vi "ArduinoSerialReadWrite.vi"(9 "LED":bool[](array[boolean])=[FALSE, FALSE, FALSE, FALSE, FALSE], 11 "VISA resource name":refnum<visa-resource-name>) -> (0 "error out":errorcluster, 1 "AIs":dbl[](array[numeric]), 2 "Buttons":bool[](array[boolean]), 3 "VISA resource name out":refnum<visa-resource-name>)   [LabVIEW 2014]
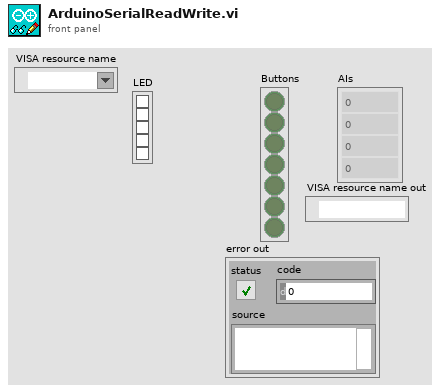
[diagram p1: front panel]
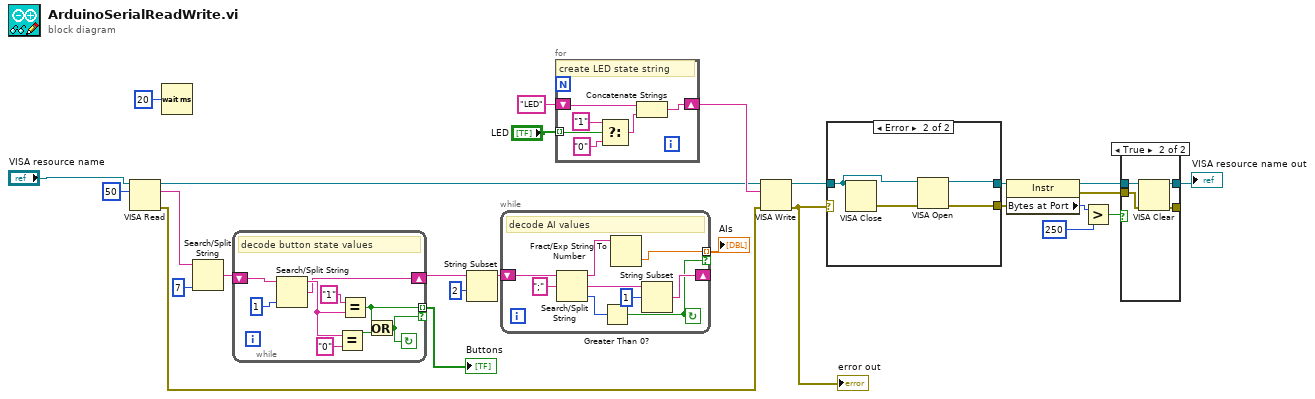
[diagram p0: block diagram]
diagram:
  n1 = VISA Read(VISA resource name="VISA resource name", byte count=u32 50) -> (VISA resource name out=w19:refnum<visa-resource-name>, read buffer=w24:string, error out=w23:errorcluster)  [unwired: 1 in, 1 out]
  n2 = Wait (ms)(milliseconds to wait=u32 20) -> ()  [unwired: 1 out]
  n3 = Search/Split String(string=w24, offset (0)=7) -> (match + rest of string=w16:string)  [unwired: 1 in, 2 out]
  n4 = while {
    tunnel: [w30] -> w15 mode=indexing if=w29
    shift-right: [w27] -> w14
    shift-left: w16 -> [w35]
    stop <- w29 continue-if-true
    # "decode button state values"
    n5 = Search/Split String(string=w35, offset (0)=1 ("length (rest)")) -> (substring before match=w28:string, match + rest of string=w27:string)  [unwired: 1 in, 1 out]
    n6 = Equal?(x=w28, y="0") -> (x = y?=w31:bool)
    n7 = Equal?(x="1" ("y"), y=w28) -> (x = y?=w30:bool)
    n8 = Or(x=w30, y=w31) -> (x .or. y?=w29:bool)
  }
  "Buttons" <- w15
  n9 = String Subset(string=w14, offset (0)=2) -> (substring=w13:string)  [unwired: 1 in]
  n10 = while {
    shift-right: [w42] -> _
    shift-left: w13 -> [w44]
    tunnel: [w38] -> w17 mode=indexing if=w37
    stop <- w37 continue-if-true
    # "decode AI values"
    n11 = Search/Split String(string=w44, search string/char (-)=";") -> (substring before match=w36:string, match + rest of string=w41:string, offset of match=w39:i32)  [unwired: 1 in]
    n12 = Greater Than 0?(x=w39) -> (x > 0?=w37:bool)
    n13 = Fract/Exp String To Number(string=w36) -> (number=w38:dbl)  [unwired: 3 in, 1 out]
    n14 = String Subset(string=w41, offset (0)=1) -> (substring=w42:string)  [unwired: 1 in]
  }
  "AIs" <- w17
  n15 = for {
    tunnel: "LED" -> [w48] mode=indexing
    shift-right: [w49] -> w20
    shift-left: "LED" -> [w50]
    # "create LED state string"
    n16 = Select(t="1", s=w48, f="0") -> (s? t:f=w47:string)
    n17 = Concatenate Strings(w50, w47) -> (w49:string)
  }
  n18 = VISA Write(VISA resource name=w19, write buffer=w20, error in (no error)=w23) -> (VISA resource name out=w9:refnum<visa-resource-name>, error out=w10:errorcluster)  [unwired: 1 out]
  "error out" <- w10
  n19 = case shown="Error" w10 {
    selector: w10 -> [w51 _]
    tunnel: [w52 w54] -> w8
    tunnel: w9 -> [w52 w55]
    tunnel: [w51 w53] -> w1
    frame No Error {
    }
    frame Error {
      n20 = VISA Close(VISA resource name=w55) -> (error out=w56:errorcluster)  [unwired: 1 in]
      n21 = VISA Open(error in (no error)=w56, VISA resource name=w55) -> (VISA resource name=w54:refnum<visa-resource-name>, error out=w53:errorcluster)  [unwired: 3 in]
    }
  }
  n22 = property class="Instr"(reference=w8, error in=w1) -> (reference out=w6:refnum<visa-resource-name>, error out=w2:errorcluster, "Bytes at Port"=w5:u32)
  n23 = Greater?(x=w5, y=u32 250) -> (0:w3:bool)
  n24 = case shown="True" w3 {
    tunnel: [w58 w62] -> w7
    tunnel: w6 -> [w58 w61]
    tunnel: w2 -> [w57 w59]
    tunnel: [w57 w60] -> _
    frame False {
    }
    frame True {
      n25 = VISA Clear(VISA resource name=w61, error in (no error)=w59) -> (VISA resource name out=w62:refnum<visa-resource-name>, error out=w60:errorcluster)
    }
  }
  "VISA resource name out" <- w7
